vi "test Rx Duration.vi"(8 "error in (no error)":errorcluster, 11 "TestCase in":refnum<class "Performance Tests.lvclass">=refnum) -> (0 "error out":errorcluster, 3 "TestCase out":refnum<class "Performance Tests.lvclass">)   [LabVIEW 2021, in "Performance Tests.lvclass"]
uses:
  Performance Tests.lvclass
  Classes/Performance/Performance.lvclass
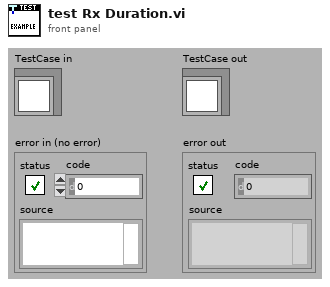
[diagram p1: front panel]
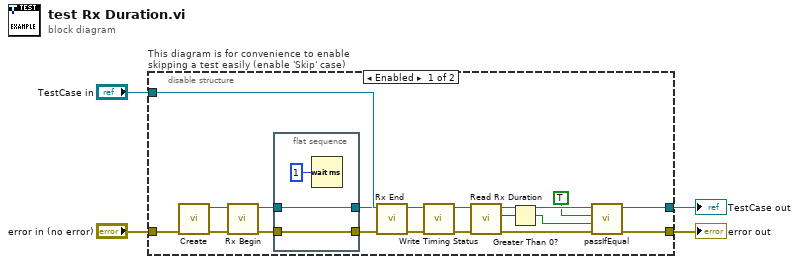
[diagram p0: block diagram]
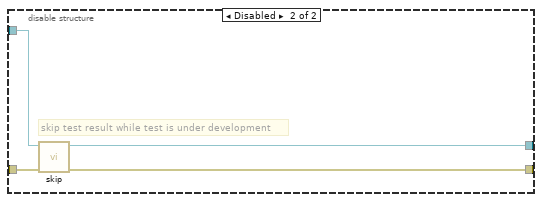
[diagram p2: hidden frame]
diagram:
  n1 = disable-structure "This diagram is for convenience to enable skipping a test easily (enable 'Skip' case)" shown="Enabled" {
    disable-tunnel: "TestCase in" -> [w21 w29]
    disable-tunnel: [w20 w27] -> w1
    disable-tunnel: [w22 w28] -> w3
    disable-tunnel: "error in (no error)" -> [w19 w26]
    frame Enabled {
      n2 = call "Create.vi"("error in (no error)"=w19) -> ("error out"=w18:errorcluster, "performance"=w17:refnum<class "Performance.lvclass">)  [unwired: 9 in]
      n3 = call "Rx Begin.vi"("error in (no error)"=w18, "Performance in"=w17) -> ("error out"=w15:errorcluster, "Performance out"=w14:refnum<class "Performance.lvclass">)  [unwired: 8 in]
      n4 = flat-sequence {
        tunnel: w15 -> [w24]
        tunnel: w14 -> [w25]
        tunnel: [w25] -> w13
        tunnel: [w24] -> w12
        frame #0 {
          n5 = Wait (ms)(milliseconds to wait=u32 1) -> ()  [unwired: 1 out]
        }
      }
      n6 = call "Rx End.vi"("error in (no error)"=w12, "Performance in"=w13) -> ("error out"=w9:errorcluster, "Performance out"=w10:refnum<class "Performance.lvclass">)  [unwired: 8 in]
      n7 = call "Write Timing Status.vi"("error in"=w9, "framework performance in"=w10) -> ("error out"=w7:errorcluster, "framework performance out"=w8:refnum<class "Performance.lvclass">)  [unwired: 8 in]
      n8 = call "Read Rx Duration.vi"("error in (no error)"=w7, "Framework Performance in"=w8) -> ("error out"=w16:errorcluster, "rx duration"=w11:u32)  [unwired: 7 in, 1 out]
      n9 = Greater Than 0?(x=w11) -> (x > 0?=w6:bool)
      n10 = call-dynamic "passIfEqual.vi"("error in (no error)"=w16, "y"=w6, "x"=TRUE, "TestCase in"=w21) -> ("error out"=w22:errorcluster, "TestCase out"=w20:refnum<class "Performance Tests.lvclass">)  [unwired: 6 in]
    }
    frame Disabled {
      # "skip test result while test is under development"
      n11 = call <vilib>:"skip.vi"("error in (no error)"=w26, "TestCase in"=w29) -> ("error out"=w28:errorcluster, "TestCase out"=w27:refnum<class "Performance Tests.lvclass">)  [unwired: 8 in]
    }
  }
  "error out" <- w3
  "TestCase out" <- w1
